vi "PH_Countdown-Counter.destructor.vi"(0 "i ref in":refnum<vi>, 5 "error in(no error)":errorcluster) -> (19 "error out":errorcluster)   [LabVIEW 2014, in "PH_Countdown-Counter.lvlib"]
doc: "This is the destructor of a class.\n\nLicense Agreement for this software:\n\nCopyright (C)\nGesellschaft für Schwerionenforschung, GSI\nPlanckstr. 1\n64291 Darmstadt\nGermany\n\nContact: D.Beck@gsi.de \n\nThis program is free software; you can redistribute it and/or modify it under the terms of the \nGNU General Public License as published by the Free Software Foundation; either version 2 of \nthe license, or (at your option) any later version.\n\nThis program is distributed in the hope that it will be useful, but WITHOUT ANY WARRANTY; \nwithout even the implied warranty of MERCHANTABILITY or FITNESS FOR A PARTICULAR PURPOSE. See the GNU General License for more details (http://www.gnu.org).\n\nGesellschaft für Schwerionenforschung, GSI\nPlanckstr. 1, 64291 Darmstadt, Germany\nFor all questions and ideas contact: M.Richter@gsi.de, H.Brand@gsi.de or D.Beck@gsi.de.\nLast update: 16-JUN-2004"
uses:
  PH_Countdown-Counter.lvlib
  CSlibraries-extern/DimLVEvent/LVDimInterface/LVDimInterface.lvlib
  PH_Basics/PH_Class/PH_Class.lvlib
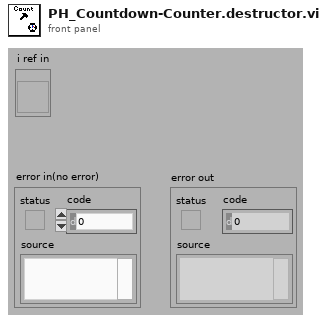
[diagram p1: front panel]
types:
  T1 = enum16{"SetAttribute", "GetAttribute", "CreateAttribute", "DestroyAttribute", "DestroyAllAtributes"}
  T2 = typedef "PH_Countdown-Counter.lvlib/PH_Countdown-Counter.i attribute.ctl" = cluster{"Machine Time":cluster{"Tag":string, "Wating Time [s]":dbl, "not linked?":bool}[], "Last Shot":cluster{"Tag":string, "Shot Time [s]":timestamp, "not linked?":bool}[], "Time since last Shot?":bool, "Calculation":cluster{"Time between Shots [s]":dbl, "Ref Remaining Time":refnum<vi>, "Service ID":i32, "over?":bool, "Ref Time between Shots":refnum<vi>, "Ref Set Mode":refnum<vi>}, "Sound?":bool, "Reminder":cluster{"# 1":cluster{"Pretime [s]":dbl, "Aktive?":bool, "Over?":bool}, "# 2":cluster{"Pretime [s]":dbl, "Aktive?":bool, "Over?":bool}}, "MainAmp only":cluster{"State":bool, "GUI Ref":refnum<vi>}}
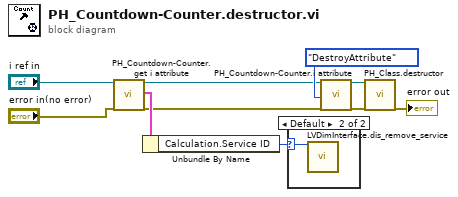
[diagram p0: block diagram]
diagram:
  n1 = call "PH_Countdown-Counter.get i attribute.vi"("i ref in"="i ref in", "error in (no error)"="error in(no error)") -> ("i ref out"=w3:refnum<vi>, "i attribute"=w9:T2, "error out"=w2:errorcluster)  [unwired: 15 in]
  n2 = Unbundle By Name(w9) -> ("Calculation.Service ID"=w4:i32)
  n3 = case shown="Default" w4 {
    selector: w4 -> [_ w11]
    frame -1 {
    }
    frame Default {
      n4 = call "LVDimInterface.dis_remove_service.vi"("my_serviceID"=w11) -> ()  [unwired: 18 in, 1 out]
    }
  }
  n5 = call "PH_Countdown-Counter.i attribute.vi"("VI Refnum"=w3, "Action"=T1."DestroyAttribute", "error in (no error)"=w2) -> ("VI Refnum out"=w7:refnum<vi>, "error out"=w8:errorcluster)  [unwired: 14 in, 1 out]
  n6 = call "PH_Class.destructor.vi"("i ref in"=w7, "error in(no error)"=w8) -> ("error out"=→"error out":errorcluster)  [unwired: 17 in]
